vi "Read_Problem.vi"(8 "error in (no error)":errorcluster) -> (0 "error out":errorcluster, 2 "Machines":u16[][](array[numeric]), 3 "Processing Times":u16[][](array[numeric]))   [LabVIEW 2013, in "OSSP_Problem.lvclass"]
uses:
  OSSP_Problem.lvclass
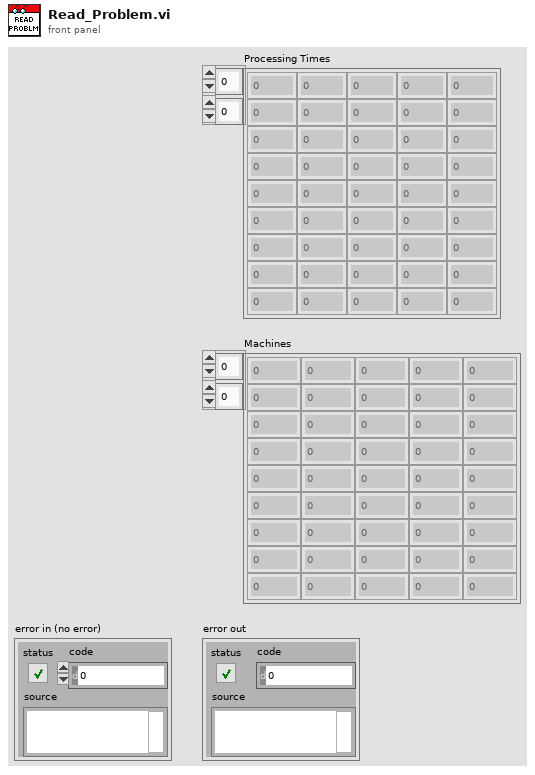
[diagram p1: front panel]
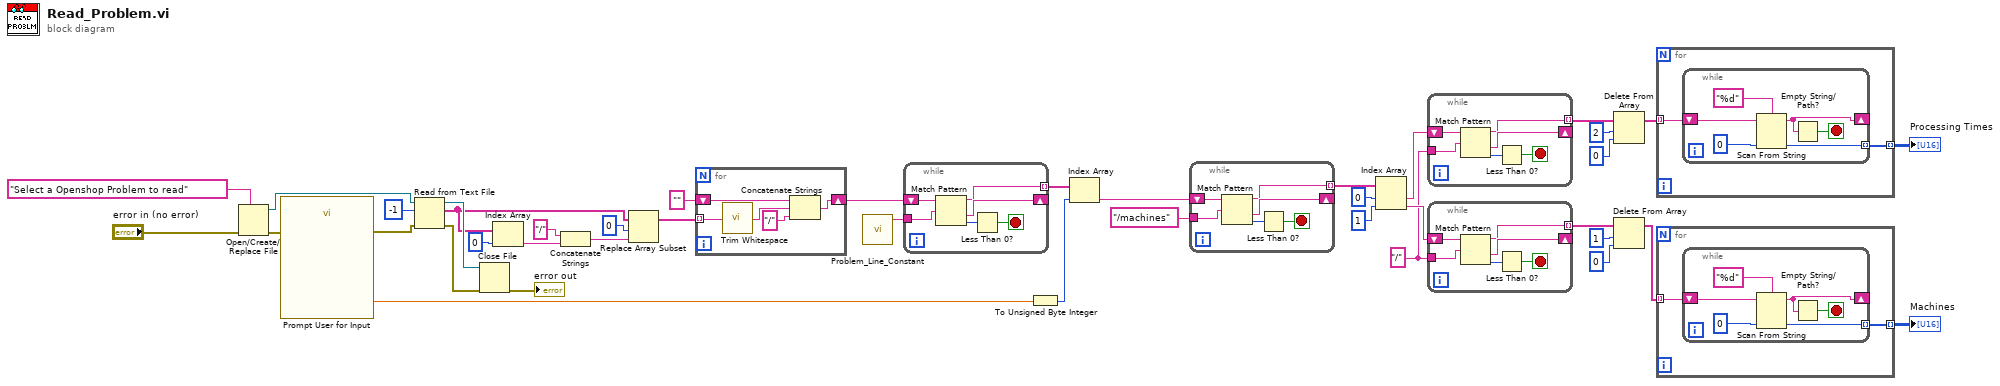
[diagram p0: block diagram]
diagram:
  w8 = "/" ("Problem Line")
  n1 = Open/Create/Replace File(error in="error in (no error)", prompt="Select a Openshop Problem to read") -> (refnum out=w37:refnum<file>, error out=w33:errorcluster)  [unwired: 4 in, 1 out]
  n2 = call "Prompt User for Input"("error in (no error)"=w33) -> ("Instance Number"=w31:dbl, "error out"=w32:errorcluster)  [unwired: 16 in, 1 out]
  n3 = Read from Text File(file (use dialog)=w37, count=-1, error in=w32) -> (refnum out=w35:refnum<file>, text=w26:string[], error out=w34:errorcluster)  [unwired: 1 in, 1 out]
  n4 = Close File(refnum=w35, error in=w34) -> (error out=→"error out":errorcluster)  [unwired: 1 out]
  n5 = Index Array(array=w26, index=0) -> (element=w29:string)
  n6 = Concatenate Strings("/" ("string"), w29) -> (w25:string)
  n7 = Replace Array Subset(array=w26, new element=w25, index=0) -> (w24:string[])
  n8 = for {
    tunnel: w24 -> [w45] mode=indexing
    shift-right: [w41] -> w22
    shift-left: "" -> [w44]
    n9 = call <vilib>:"Trim Whitespace.vi"("string"=w45) -> ("trimmed string"=w43:string)  [unwired: 1 in]
    n10 = Concatenate Strings(w44, w43, "/" ("string")) -> (w41:string)
  }
  n11 = call "Problem_Line_Constant.vi"() -> ("Problem Line"=w21:string)  [unwired: 11 in]
  n12 = while {
    tunnel: w21 -> [w50]
    shift-right: [w48] -> _
    shift-left: w22 -> [w51]
    tunnel: [w47] -> w20 mode=indexing
    stop <- w46 stop-if-true
    n13 = Match Pattern(string=w51, regular expression=w50) -> (before substring=w47:string, after substring=w48:string, offset past match=w49:i32)  [unwired: 1 in, 1 out]
    n14 = Less Than 0?(x=w49) -> (x < 0?=w46:bool)
  }
  n15 = To Unsigned Byte Integer(number=w31) -> (unsigned 8bit integer=w19:u8)
  n16 = Index Array(array=w20, index=w19) -> (element=w18:string)
  n17 = while {
    tunnel: "/machines" ("Problem Line") -> [w56]
    shift-right: [w54] -> _
    shift-left: w18 -> [w57]
    tunnel: [w53] -> w16 mode=indexing
    stop <- w52 stop-if-true
    n18 = Match Pattern(string=w57, regular expression=w56) -> (before substring=w53:string, after substring=w54:string, offset past match=w55:i32)  [unwired: 1 in, 1 out]
    n19 = Less Than 0?(x=w55) -> (x < 0?=w52:bool)
  }
  n20 = Index Array(array=w16, index #1=0 ("index"), index #2=1 ("index")) -> (element #1=w14:string, element #2=w9:string)
  n21 = while {
    tunnel: w8 -> [w62]
    shift-right: [w60] -> _
    shift-left: w14 -> [w63]
    tunnel: [w59] -> w13 mode=indexing
    stop <- w58 stop-if-true
    n22 = Match Pattern(string=w63, regular expression=w62) -> (before substring=w59:string, after substring=w60:string, offset past match=w61:i32)  [unwired: 1 in, 1 out]
    n23 = Less Than 0?(x=w61) -> (x < 0?=w58:bool)
  }
  n24 = while {
    tunnel: w8 -> [w68]
    shift-right: [w66] -> _
    shift-left: w9 -> [w69]
    tunnel: [w65] -> w7 mode=indexing
    stop <- w64 stop-if-true
    n25 = Match Pattern(string=w69, regular expression=w68) -> (before substring=w65:string, after substring=w66:string, offset past match=w67:i32)  [unwired: 1 in, 1 out]
    n26 = Less Than 0?(x=w67) -> (x < 0?=w64:bool)
  }
  n27 = Delete From Array(array=w13, length=2, index=0) -> (array with subset deleted=w4:string[])  [unwired: 1 out]
  n28 = Delete From Array(array=w7, length=1, index=0) -> (array with subset deleted=w2:string[])  [unwired: 1 out]
  n29 = for {
    tunnel: w4 -> [w71] mode=indexing
    tunnel: [w70] -> w3 mode=indexing
    n30 = while {
      shift-right: [w73] -> _
      shift-left: w71 -> [w77]
      tunnel: [w75] -> w70 mode=indexing
      stop <- w72 stop-if-true
      n31 = Scan From String(format string="%d", input string=w77, default 1=u16 0 ("default value 1")) -> (remaining string=w73:string, output 1=w75:u16)  [unwired: 2 in, 2 out]
      n32 = Empty String/Path?(string/path=w73) -> (empty?=w72:bool)
    }
  }
  "Processing Times" <- w3
  n33 = for {
    tunnel: w2 -> [w79] mode=indexing
    tunnel: [w78] -> w1 mode=indexing
    n34 = while {
      shift-right: [w81] -> _
      shift-left: w79 -> [w85]
      tunnel: [w83] -> w78 mode=indexing
      stop <- w80 stop-if-true
      n35 = Scan From String(format string="%d", input string=w85, default 1=u16 0 ("default value 1")) -> (remaining string=w81:string, output 1=w83:u16)  [unwired: 2 in, 2 out]
      n36 = Empty String/Path?(string/path=w81) -> (empty?=w80:bool)
    }
  }
  "Machines" <- w1
